vi "Arm Control Teleop.vi"(11 "Controller Mode":enum16{"X-Box Controller", "Joysticks"}(ring)) -> (3 "Motor Output":dbl)   [LabVIEW 2015]
uses:
  Robot Global Data.vi
  <vilib>/Rock Robotics/WPI/Utilities/WPI_GetSetVariantRefNum.vi
panel:
  in  "Upper Switch Pressed":bool
  in  "Lower Switch Pressed":bool
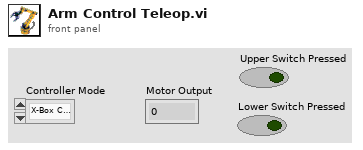
[diagram p1: front panel]
types:
  T1 = typedef "WPI_SwitchDevRef.ctl" = cluster{"DevStatus":errorcluster, "DIO Channel":T2, "CntIndex":T3, "Normally Closed":bool}
  T2 = typedef "FPGA_DIOChannel.ctl" = enum8{"DIO 0", "DIO 1", "DIO 2", "DIO 3", "DIO 4", "DIO 5", "DIO 6", "DIO 7", "DIO 8", "DIO 9", "DIO MXP 0", "DIO MXP 1", "DIO MXP 2", "DIO MXP 3", "DIO MXP 4", "DIO MXP 5", "DIO MXP 6", "DIO MXP 7", "DIO MXP 8", "DIO MXP 9", "DIO MXP 10", "DIO MXP 11", "DIO MXP 12", "DIO MXP 13", "DIO MXP 14", "DIO MXP 15", "Invalid"}
  T3 = typedef "FPGA_CounterCtrSystemIndex.ctl" = enum8{"Ctr 0", "Ctr 1", "Ctr 2", "Ctr 3", "Ctr 4", "Ctr 5", "Ctr 6", "Ctr 7", "Invalid"}
  T4 = typedef "WPI_JoystickDevRef.ctl" = cluster{"Device":T5}
  T5 = typedef "WPI_JoystickDeviceEnum.ctl" = enum16{"USB 0", "USB 1", "USB 2", "USB 3", "USB 4", "USB 5"}
  T6 = typedef "WPI_MotorControlDeviceRef.ctl" = cluster{"DeviceStatus":errorcluster, "Type":T7, "PWM":cluster{"PWM Channel":T8, "DeadBand":T9}, "CAN":cluster{"Device Number":u8, "Control Mode":T10, "Semaphore":T11, "Max Vout":dbl, "TalonSRX Control Mode":T12}, "Invert":bool}
  T7 = typedef "WPI_MotorControlType.ctl" = enum16{"PWM", "CAN", "CANTalonSRX"}
  T8 = typedef "FPGA_DIOPWMChannel.ctl" = enum8{"PWM 0", "PWM 1", "PWM 2", "PWM 3", "PWM 4", "PWM 5", "PWM 6", "PWM 7", "PWM 8", "PWM 9", "PWM MXP 0", "PWM MXP 1", "PWM MXP 2", "PWM MXP 3", "PWM MXP 4", "PWM MXP 5", "PWM MXP 6", "PWM MXP 7", "PWM MXP 8", "PWM MXP 9", "Invalid"}
  T9 = typedef "WPI_PWMDeadband.ctl" = cluster{"Name":string, "maxPositivePwm":i32, "minPositivePwm":i32, "centerPwm":i32, "maxNegativePwm":i32, "minNegativePwm":i32, "angularRange":u16}
  T10 = typedef "WPI_CANJaguar_ControlMode.ctl" = enum8{"Percent VBus", "Current", "Speed", "Position", "Voltage"}
  T11 = typedef "Semaphore RefNum" = refnum<k1>
  T12 = typedef "WPI_CANTalonSRX_APIControlMode.ctl" = enum8{"Percent VBus", "Speed", "Position", "Slave", "Unchanged / Invalid", "Voltage Compensation", "Current", "Motion Profile"}
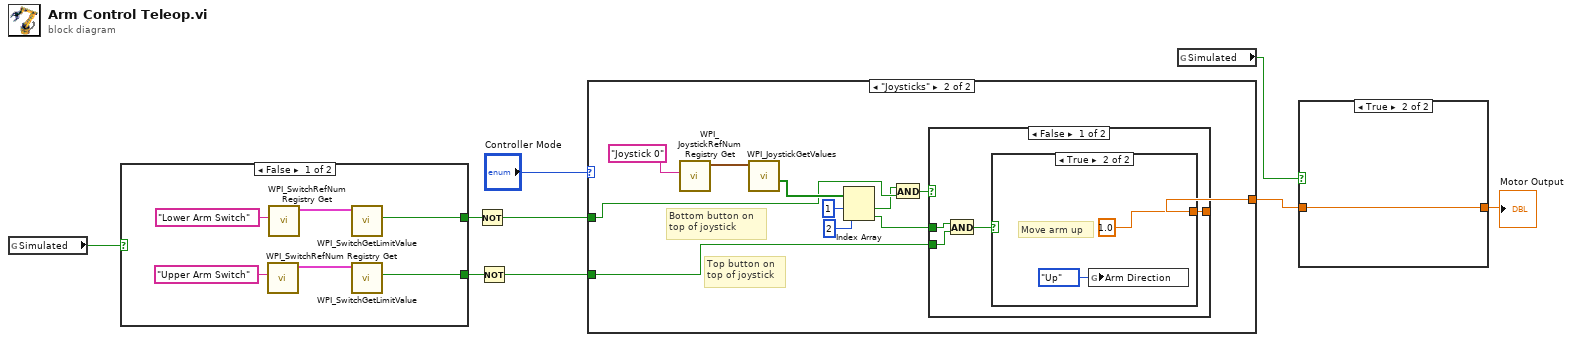
[diagram p0: block diagram]
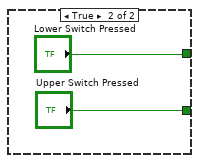
[diagram p2: hidden frame]
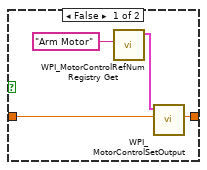
[diagram p3: hidden frame]
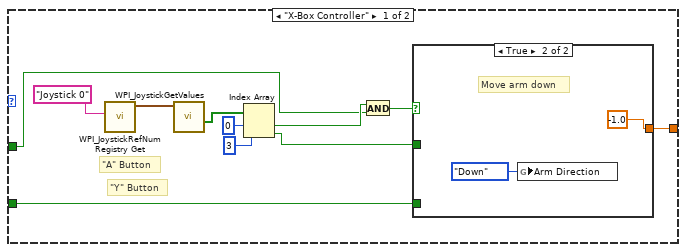
[diagram p4: hidden frame]
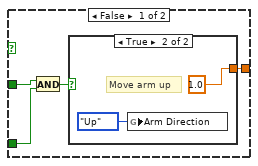
[diagram p5: hidden frame]
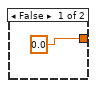
[diagram p6: hidden frame]
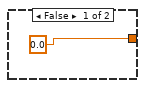
[diagram p7: hidden frame]
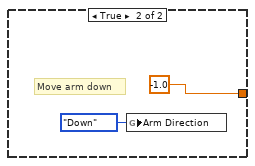
[diagram p8: hidden frame]
diagram:
  n1 = global read "Robot Global Data.vi" "Simulated"() -> (w2:bool)
  n2 = case shown="False" w2 {
    tunnel: [w11 "Lower Switch Pressed"] -> w1
    tunnel: [w10 "Upper Switch Pressed"] -> w5
    frame False {
      n3 = call <vilib>:"WPI_SwitchRefNum Registry Get.vi"("refnum name"="Upper Arm Switch") -> ("SwitchDevRef"=w13:T1)  [unwired: 9 in, 1 out]
      n4 = call <vilib>:"WPI_SwitchRefNum Registry Get.vi"("refnum name"="Lower Arm Switch") -> ("SwitchDevRef"=w12:T1)  [unwired: 9 in, 1 out]
      n5 = call <vilib>:"WPI_SwitchGetLimitValue.vi"("SwitchDevRef"=w12) -> ("Switch Pressed"=w11:bool)  [unwired: 8 in, 2 out]
      n6 = call <vilib>:"WPI_SwitchGetLimitValue.vi"("SwitchDevRef"=w13) -> ("Switch Pressed"=w10:bool)  [unwired: 8 in, 2 out]
    }
    frame True {
    }
  }
  n7 = Not(x=w1) -> (.not. x?=w4:bool)
  n8 = Not(x=w5) -> (.not. x?=w3:bool)
  n9 = case shown="\"Joysticks\"" "Controller Mode" {
    tunnel: [w22 w42] -> w8
    tunnel: w4 -> [w18 w40]
    tunnel: w3 -> [w19 w38]
    frame "X-Box Controller" {
      # "\"Y\" Button"
      # "\"A\" Button"
      n10 = call <vilib>:"WPI_JoystickRefNum Registry Get.vi"("refnum name"="Joystick 0") -> ("JoystickDevRef"=w27:T4)  [unwired: 9 in, 1 out]
      n11 = call <vilib>:"WPI_JoystickGetValues.vi"("JoystickDevRef"=w27) -> ("Buttons"=w26:bool[])  [unwired: 6 in, 4 out]
      n12 = Index Array(array=w26, index #1=0 ("index"), index #2=3 ("index")) -> (element #1=w20:bool, element #2=w23:bool)
      n13 = And(x=w20, y=w18) -> (x .and. y?=w21:bool)
      n14 = case shown="True" w21 {
        tunnel: w23 -> [w30 _]
        tunnel: [w32 -1.0] -> w22
        tunnel: w19 -> [w29 _]
        frame False {
          n15 = And(x=w30, y=w29) -> (x .and. y?=w31:bool)
          n16 = case shown="True" w31 {
            tunnel: [0.0 1.0] -> w32
            frame False {
            }
            frame True {
              # "Move arm up"
              n17 = global write "Robot Global Data.vi" "Arm Direction"(enum16{"Up", "Down"}."Up" ("Arm Direction")) -> ()
            }
          }
        }
        frame True {
          # "Move arm down"
          n18 = global write "Robot Global Data.vi" "Arm Direction"(enum16{"Up", "Down"}."Down" ("Arm Direction")) -> ()
        }
      }
    }
    frame "Joysticks" {
      # "Top button on\ntop of joystick"
      # "Bottom button on\ntop of joystick"
      n19 = call <vilib>:"WPI_JoystickRefNum Registry Get.vi"("refnum name"="Joystick 0") -> ("JoystickDevRef"=w47:T4)  [unwired: 9 in, 1 out]
      n20 = call <vilib>:"WPI_JoystickGetValues.vi"("JoystickDevRef"=w47) -> ("Buttons"=w43:bool[])  [unwired: 6 in, 4 out]
      n21 = Index Array(array=w43, index #1=1 ("index"), index #2=2 ("index")) -> (element #1=w39:bool, element #2=w44:bool)
      n22 = And(x=w39, y=w40) -> (x .and. y?=w41:bool)
      n23 = case shown="False" w41 {
        tunnel: w44 -> [w49 _]
        tunnel: [w52 -1.0] -> w42
        tunnel: w38 -> [w50 _]
        frame False {
          n24 = And(x=w49, y=w50) -> (x .and. y?=w51:bool)
          n25 = case shown="True" w51 {
            tunnel: [0.0 1.0] -> w52
            frame False {
            }
            frame True {
              # "Move arm up"
              n26 = global write "Robot Global Data.vi" "Arm Direction"(enum16{"Up", "Down"}."Up" ("Arm Direction")) -> ()
            }
          }
        }
        frame True {
          # "Move arm down"
          n27 = global write "Robot Global Data.vi" "Arm Direction"(enum16{"Up", "Down"}."Down" ("Arm Direction")) -> ()
        }
      }
    }
  }
  n28 = global read "Robot Global Data.vi" "Simulated"() -> (w6:bool)
  n29 = case shown="True" w6 {
    tunnel: [w61 w62] -> w9
    tunnel: w8 -> [w59 w62]
    frame False {
      n30 = call <vilib>:"WPI_MotorControlRefNum Registry Get.vi"("refnum name"="Arm Motor") -> ("MotorControlDevRef"=w60:T6)  [unwired: 9 in, 1 out]
      n31 = call <vilib>:"WPI_MotorControlSetOutput.vi"("Output"=w59, "MotorControlDevRef"=w60) -> ("Motor Output"=w61:dbl)  [unwired: 7 in, 2 out]
    }
    frame True {
    }
  }
  "Motor Output" <- w9
